vi "Arduino read multiple frequencies.vi"(7 "openQCM gate time":i32, 8 "arduino addresses in":T1, 11 "arduinos on?":bool) -> (0 "arduino addresses out":T1, 1 "openQCM frequencies out":T2, 3 "arduinos on":bool)   [LabVIEW 2014]
uses:
  <vilib>/Analysis/baseanly.llb/Mean (DBL).vi
  <vilib>/Analysis/NI_AALBase.lvlib
panel:
  out "Temp (K) 6":dbl
  out "Temp (K) 5":dbl
  out "Temp (K) 4":dbl
  out "Temp (K) 3":dbl
  out "Temp (K) 2":dbl
  out "Temp (K)":dbl
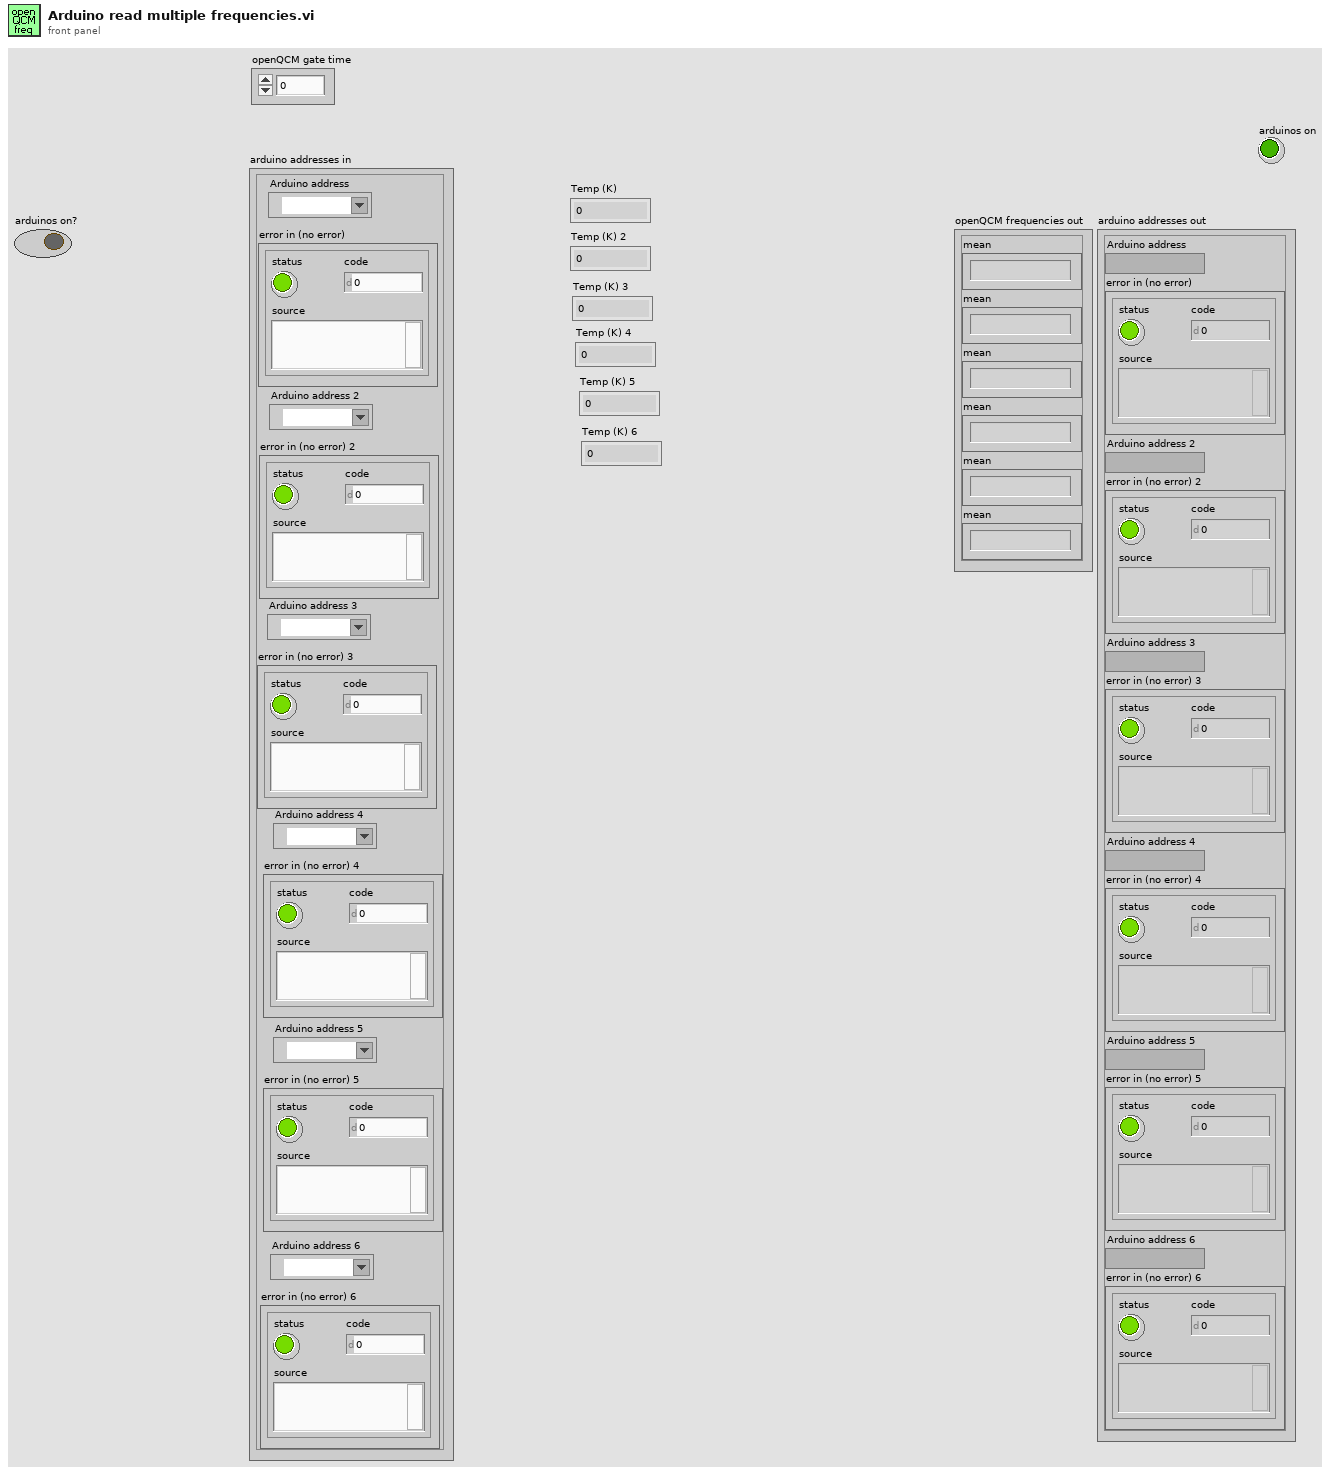
[diagram p1: front panel]
types:
  T1 = cluster{"Arduino address":refnum<visa-resource-name>, "error in (no error)":errorcluster, "Arduino address 2":refnum<visa-resource-name>, "error in (no error) 2":errorcluster, "Arduino address 3":refnum<visa-resource-name>, "error in (no error) 3":errorcluster, "Arduino address 4":refnum<visa-resource-name>, "error in (no error) 4":errorcluster, "Arduino address 5":refnum<visa-resource-name>, "error in (no error) 5":errorcluster, "Arduino address 6":refnum<visa-resource-name>, "error in (no error) 6":errorcluster}
  T2 = cluster{"mean":string, "mean":string, "mean":string, "mean":string, "mean":string, "mean":string}
  T3 = cluster{"mean":dbl, "mean":dbl, "mean":dbl, "mean":dbl, "mean":dbl, "mean":dbl}
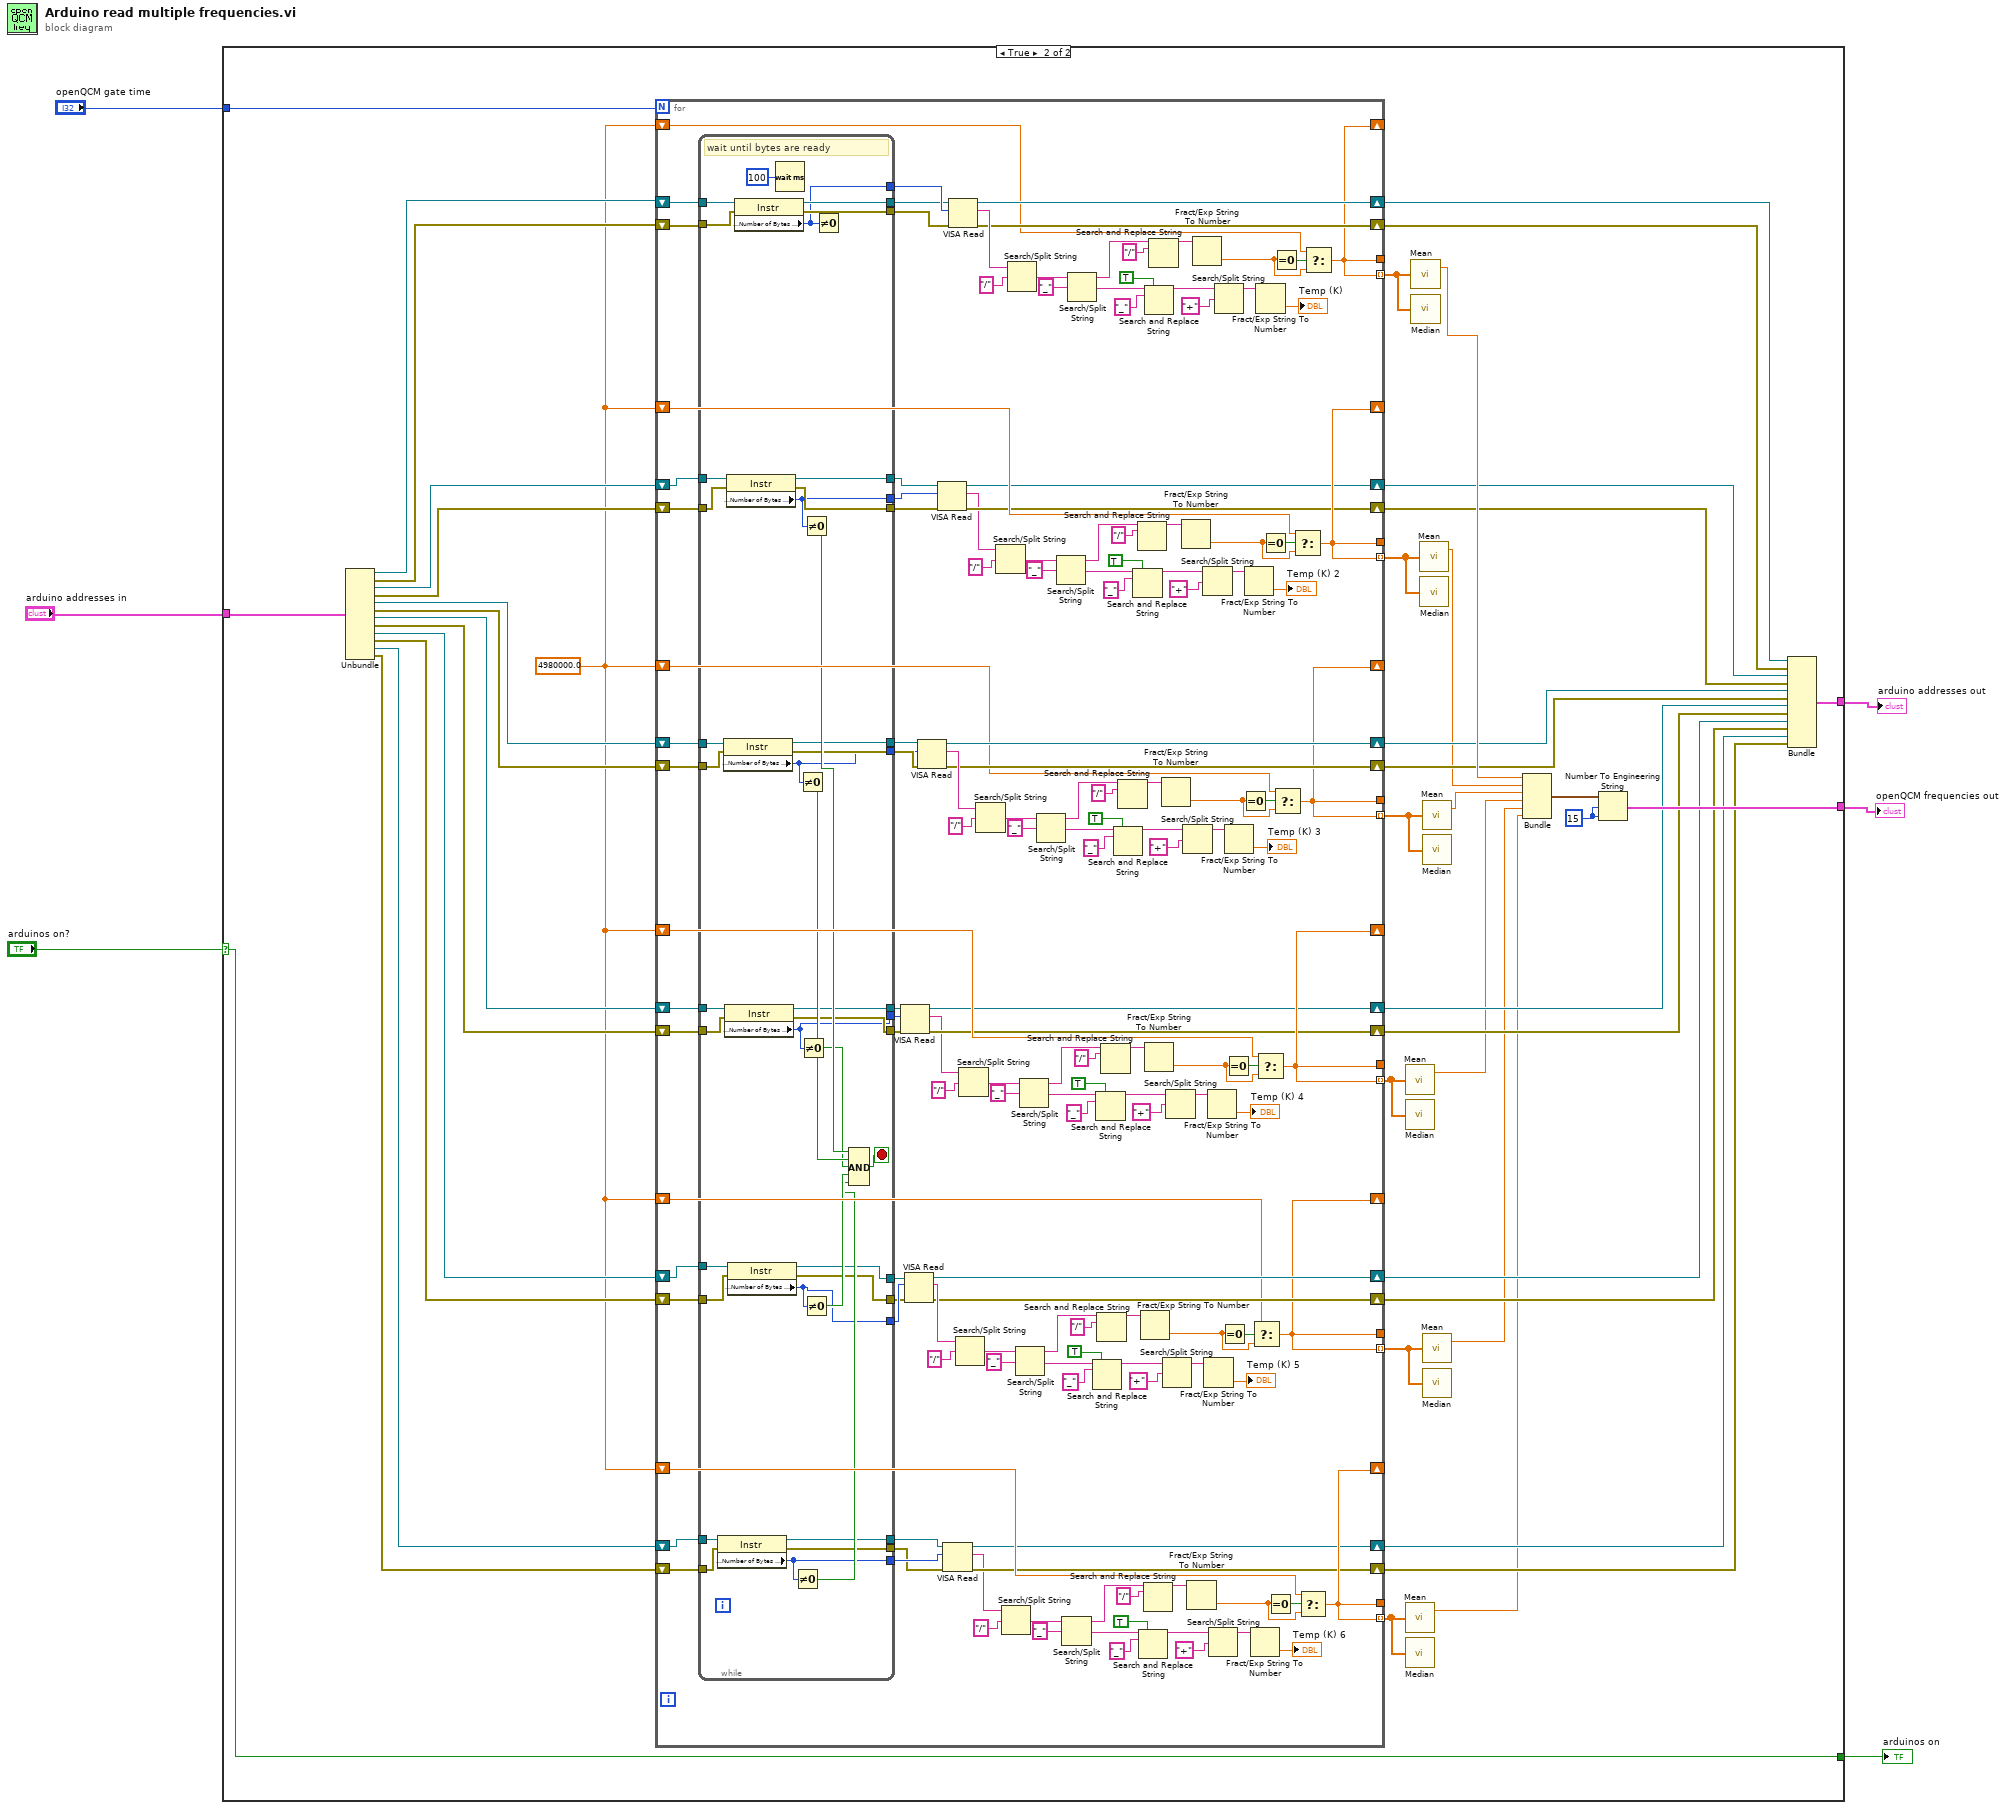
[diagram p0: block diagram]
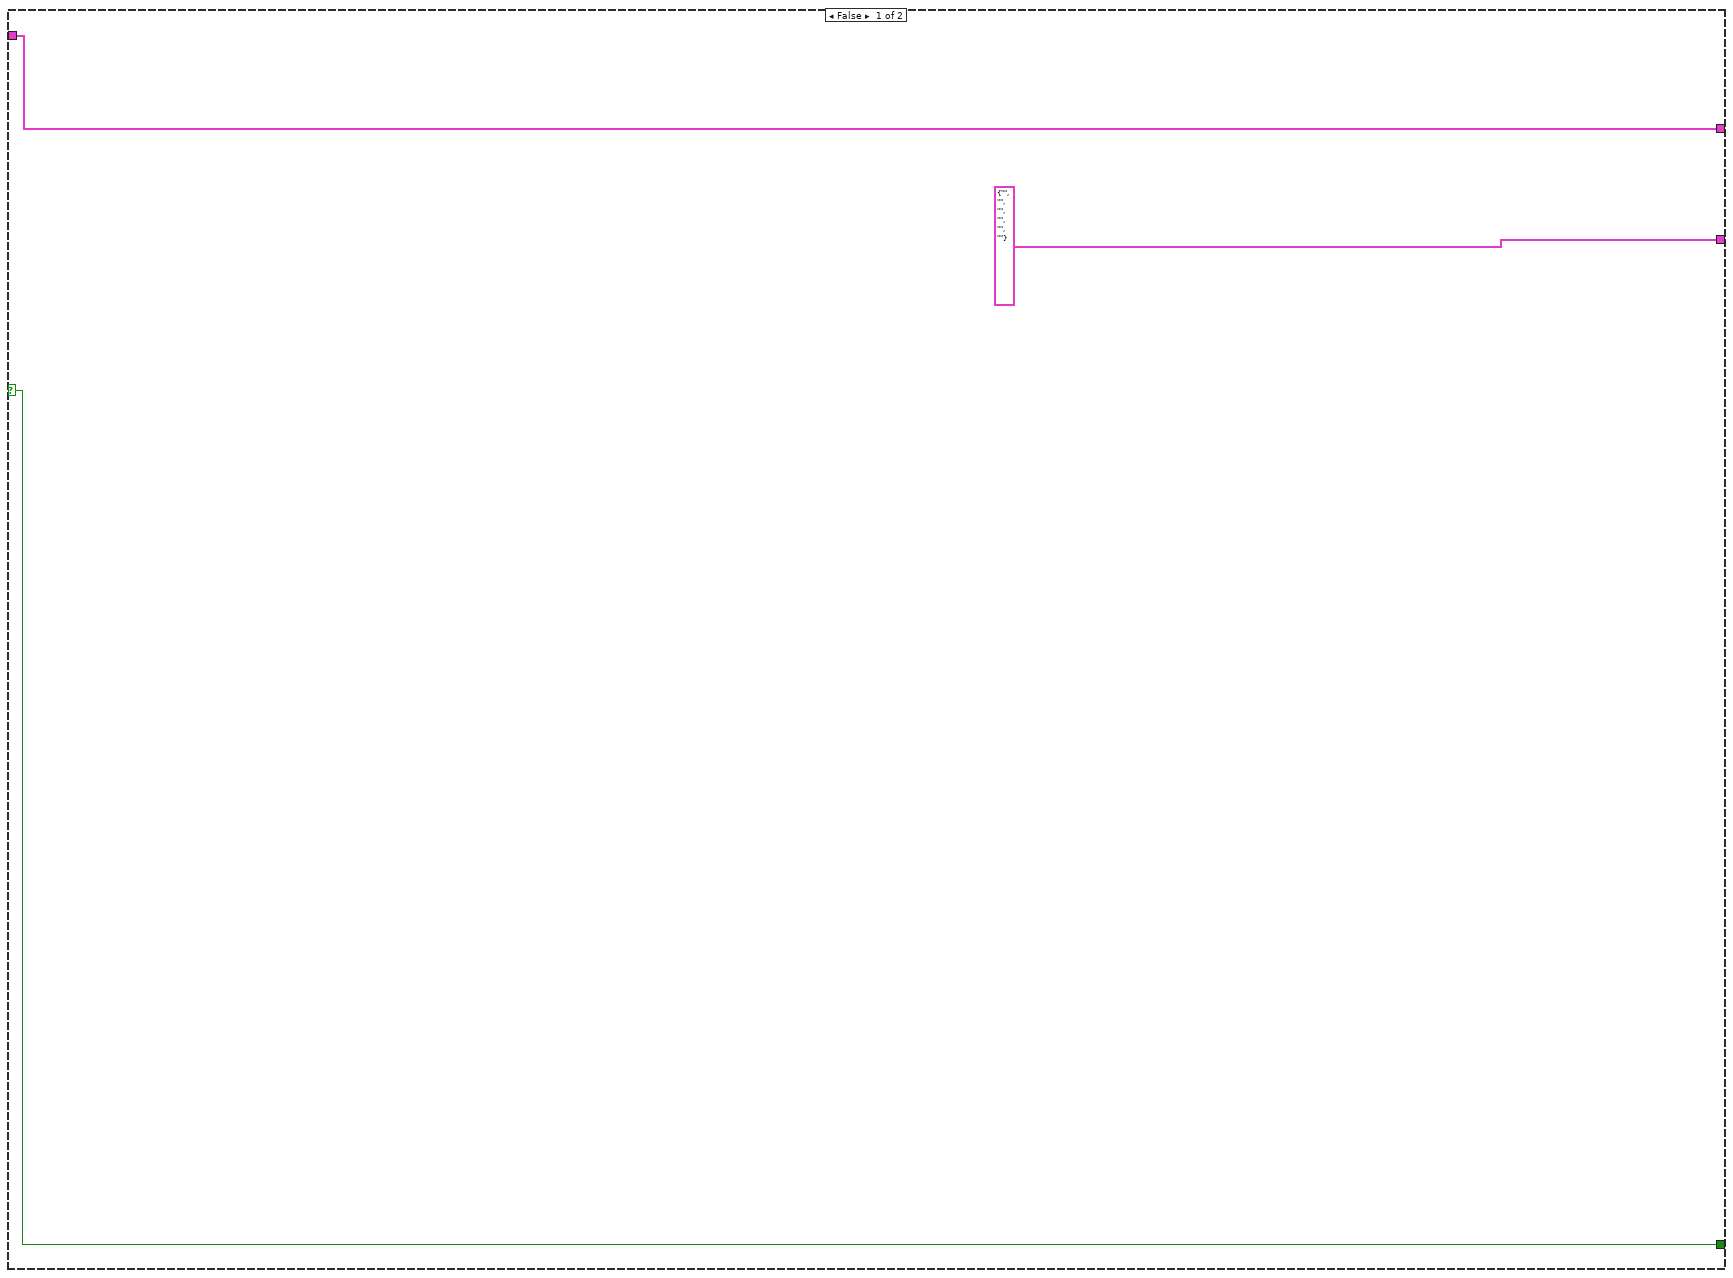
[diagram p2: hidden frame]
diagram:
  n1 = case shown="True" "arduinos on?" {
    selector: "arduinos on?" -> [w9 w10]
    tunnel: "arduino addresses in" -> [w8 w53]
    tunnel: "openQCM gate time" -> [_ w49]
    tunnel: [T2 {"mean"="", "mean"="", "mean"="", "mean"="", "mean"="", "mean"=""} w47] -> w4
    tunnel: [w8 w11] -> w3
    tunnel: [w9 w10] -> w1
    frame False {
    }
    frame True {
      w27 = 4980000.0
      w50 = i16 15 ("width (-)")
      n2 = Unbundle(w53) -> ("Arduino address"=w52:refnum<visa-resource-name>, "error in (no error)"=w51:errorcluster, "Arduino address 2"=w37:refnum<visa-resource-name>, "error in (no error) 2"=w36:errorcluster, "Arduino address 3"=w35:refnum<visa-resource-name>, "error in (no error) 3"=w34:errorcluster, "Arduino address 4"=w33:refnum<visa-resource-name>, "error in (no error) 4"=w32:errorcluster, "Arduino address 5"=w31:refnum<visa-resource-name>, "error in (no error) 5"=w28:errorcluster, "Arduino address 6"=w29:refnum<visa-resource-name>, "error in (no error) 6"=w30:errorcluster)
      n3 = for {
        N: w49 -> [_]
        tunnel: [w180] -> _
        shift-right: [w189] -> w44
        shift-left: w52 -> [w184]
        shift-right: [w188] -> w43
        shift-left: w51 -> [w183]
        tunnel: [w180] -> w48 mode=indexing
        shift-right: [w180] -> _
        shift-left: w27 -> [w179]
        tunnel: [w177] -> _
        shift-right: [w173] -> w26
        shift-left: w37 -> [w78]
        shift-right: [w174] -> w25
        shift-left: w36 -> [w77]
        tunnel: [w177] -> w42 mode=indexing
        shift-right: [w177] -> _
        shift-left: w27 -> [w178]
        tunnel: [w140] -> _
        shift-right: [w144] -> w24
        shift-left: w35 -> [w70]
        shift-right: [w143] -> w23
        shift-left: w34 -> [w69]
        tunnel: [w140] -> w41 mode=indexing
        shift-right: [w140] -> _
        shift-left: w27 -> [w139]
        tunnel: [w137] -> _
        shift-right: [w133] -> w22
        shift-left: w33 -> [w68]
        shift-right: [w134] -> w21
        shift-left: w32 -> [w67]
        tunnel: [w137] -> w40 mode=indexing
        shift-right: [w137] -> _
        shift-left: w27 -> [w138]
        tunnel: [w100] -> _
        shift-right: [w104] -> w20
        shift-left: w31 -> [w59]
        shift-right: [w103] -> w19
        shift-left: w28 -> [w58]
        tunnel: [w100] -> w39 mode=indexing
        shift-right: [w100] -> _
        shift-left: w27 -> [w99]
        tunnel: [w97] -> _
        shift-right: [w93] -> w18
        shift-left: w29 -> [w61]
        shift-right: [w94] -> w17
        shift-left: w30 -> [w60]
        tunnel: [w97] -> w38 mode=indexing
        shift-right: [w97] -> _
        shift-left: w27 -> [w98]
        n4 = while {
          tunnel: w183 -> [w239]
          tunnel: w184 -> [w240]
          tunnel: [w238] -> w182
          tunnel: [w237] -> w181
          tunnel: [w236] -> w185
          tunnel: w78 -> [w232]
          tunnel: w77 -> [w231]
          tunnel: [w230] -> w74
          tunnel: [w229] -> w75
          tunnel: [w228] -> w76
          tunnel: [w227] -> w73
          tunnel: [w226] -> w72
          tunnel: [w225] -> w71
          tunnel: w70 -> [w224]
          tunnel: w69 -> [w223]
          tunnel: w68 -> [w221]
          tunnel: w67 -> [w220]
          tunnel: [w219] -> w54
          tunnel: [w218] -> w66
          tunnel: [w217] -> w65
          tunnel: [w213] -> w64
          tunnel: [w212] -> w63
          tunnel: [w211] -> w62
          tunnel: w61 -> [w210]
          tunnel: w60 -> [w209]
          tunnel: w59 -> [w208]
          tunnel: w58 -> [w207]
          tunnel: [w205] -> w57
          tunnel: [w206] -> w56
          tunnel: [w204] -> w55
          stop <- w233 stop-if-true
          # "wait until bytes are ready"
          n5 = property class="Instr"(reference=w210, error in=w209) -> (reference out=w211:refnum<visa-resource-name>, error out=w212:errorcluster, "Serial Settings:Number of Bytes at Serial Port"=w213:u32)
          n6 = property class="Instr"(reference=w224, error in=w223) -> (reference out=w225:refnum<visa-resource-name>, error out=w227:errorcluster, "Serial Settings:Number of Bytes at Serial Port"=w226:u32)
          n7 = property class="Instr"(reference=w221, error in=w220) -> (reference out=w219:refnum<visa-resource-name>, error out=w218:errorcluster, "Serial Settings:Number of Bytes at Serial Port"=w217:u32)
          n8 = property class="Instr"(reference=w232, error in=w231) -> (reference out=w230:refnum<visa-resource-name>, error out=w229:errorcluster, "Serial Settings:Number of Bytes at Serial Port"=w228:u32)
          n9 = property class="Instr"(reference=w208, error in=w207) -> (reference out=w205:refnum<visa-resource-name>, error out=w204:errorcluster, "Serial Settings:Number of Bytes at Serial Port"=w206:u32)
          n10 = property class="Instr"(reference=w240, error in=w239) -> (reference out=w237:refnum<visa-resource-name>, error out=w238:errorcluster, "Serial Settings:Number of Bytes at Serial Port"=w236:u32)
          n11 = Wait (ms)(milliseconds to wait=u32 100) -> ()  [unwired: 1 out]
          n12 = Not Equal To 0?(x=w213) -> (x != 0?=w214:bool)
          n13 = Not Equal To 0?(x=w226) -> (x != 0?=w222:bool)
          n14 = Not Equal To 0?(x=w217) -> (x != 0?=w216:bool)
          n15 = Not Equal To 0?(x=w228) -> (x != 0?=w234:bool)
          n16 = Not Equal To 0?(x=w206) -> (x != 0?=w215:bool)
          n17 = Not Equal To 0?(x=w236) -> ()  [unwired: 1 out]
          n18 = Compound Arithmetic op=AND(w234, w222, w216, w215, w214) -> (w233:bool)
        }
        n19 = VISA Read(VISA resource name=w54, byte count=w65, error in (no error)=w66) -> (VISA resource name out=w133:refnum<visa-resource-name>, read buffer=w119:string, error out=w134:errorcluster)  [unwired: 1 out]
        n20 = VISA Read(VISA resource name=w57, byte count=w56, error in (no error)=w55) -> (VISA resource name out=w104:refnum<visa-resource-name>, read buffer=w118:string, error out=w103:errorcluster)  [unwired: 1 out]
        n21 = VISA Read(VISA resource name=w71, byte count=w72, error in (no error)=w73) -> (VISA resource name out=w144:refnum<visa-resource-name>, read buffer=w158:string, error out=w143:errorcluster)  [unwired: 1 out]
        n22 = VISA Read(VISA resource name=w74, byte count=w76, error in (no error)=w75) -> (VISA resource name out=w173:refnum<visa-resource-name>, read buffer=w159:string, error out=w174:errorcluster)  [unwired: 1 out]
        n23 = VISA Read(VISA resource name=w62, byte count=w64, error in (no error)=w63) -> (VISA resource name out=w93:refnum<visa-resource-name>, read buffer=w79:string, error out=w94:errorcluster)  [unwired: 1 out]
        n24 = VISA Read(VISA resource name=w181, byte count=w185, error in (no error)=w182) -> (VISA resource name out=w189:refnum<visa-resource-name>, read buffer=w203:string, error out=w188:errorcluster)  [unwired: 1 out]
        n25 = Search/Split String(string=w118, search string/char (-)="/") -> (match + rest of string=w110:string)  [unwired: 1 in, 2 out]
        n26 = Search/Split String(string=w119, search string/char (-)="/") -> (match + rest of string=w127:string)  [unwired: 1 in, 2 out]
        n27 = Search/Split String(string=w158, search string/char (-)="/") -> (match + rest of string=w150:string)  [unwired: 1 in, 2 out]
        n28 = Search/Split String(string=w159, search string/char (-)="/") -> (match + rest of string=w167:string)  [unwired: 1 in, 2 out]
        n29 = Search/Split String(string=w79, search string/char (-)="/") -> (match + rest of string=w87:string)  [unwired: 1 in, 2 out]
        n30 = Search/Split String(string=w203, search string/char (-)="/") -> (match + rest of string=w195:string)  [unwired: 1 in, 2 out]
        n31 = Search/Split String(string=w110, search string/char (-)="_") -> (substring before match=w116:string, match + rest of string=w111:string)  [unwired: 1 in, 1 out]
        n32 = Search/Split String(string=w127, search string/char (-)="_") -> (substring before match=w121:string, match + rest of string=w126:string)  [unwired: 1 in, 1 out]
        n33 = Search/Split String(string=w150, search string/char (-)="_") -> (substring before match=w156:string, match + rest of string=w151:string)  [unwired: 1 in, 1 out]
        n34 = Search/Split String(string=w167, search string/char (-)="_") -> (substring before match=w161:string, match + rest of string=w166:string)  [unwired: 1 in, 1 out]
        n35 = Search/Split String(string=w87, search string/char (-)="_") -> (substring before match=w81:string, match + rest of string=w86:string)  [unwired: 1 in, 1 out]
        n36 = Search/Split String(string=w195, search string/char (-)="_") -> (substring before match=w201:string, match + rest of string=w196:string)  [unwired: 1 in, 1 out]
        n37 = Search and Replace String(replace all?=TRUE ("replace all? (F)"), input string=w111, search string="_") -> (result string=w105:string)  [unwired: 5 in, 3 out]
        n38 = Search and Replace String(replace all?=TRUE ("replace all? (F)"), input string=w126, search string="_") -> (result string=w132:string)  [unwired: 5 in, 3 out]
        n39 = Search and Replace String(input string=w116, search string="/" ("replace string (\"\")")) -> (result string=w107:string)  [unwired: 6 in, 3 out]
        n40 = Search and Replace String(input string=w121, search string="/" ("replace string (\"\")")) -> (result string=w130:string)  [unwired: 6 in, 3 out]
        n41 = Search and Replace String(replace all?=TRUE ("replace all? (F)"), input string=w151, search string="_") -> (result string=w145:string)  [unwired: 5 in, 3 out]
        n42 = Search and Replace String(input string=w156, search string="/" ("replace string (\"\")")) -> (result string=w147:string)  [unwired: 6 in, 3 out]
        n43 = Search and Replace String(replace all?=TRUE ("replace all? (F)"), input string=w166, search string="_") -> (result string=w172:string)  [unwired: 5 in, 3 out]
        n44 = Search and Replace String(input string=w161, search string="/" ("replace string (\"\")")) -> (result string=w170:string)  [unwired: 6 in, 3 out]
        n45 = Search and Replace String(replace all?=TRUE ("replace all? (F)"), input string=w86, search string="_") -> (result string=w92:string)  [unwired: 5 in, 3 out]
        n46 = Fract/Exp String To Number(string=w107) -> (number=w101:dbl)  [unwired: 3 in, 1 out]
        n47 = Search and Replace String(input string=w81, search string="/" ("replace string (\"\")")) -> (result string=w90:string)  [unwired: 6 in, 3 out]
        n48 = Search and Replace String(replace all?=TRUE ("replace all? (F)"), input string=w196, search string="_") -> (result string=w190:string)  [unwired: 5 in, 3 out]
        n49 = Fract/Exp String To Number(string=w130) -> (number=w136:dbl)  [unwired: 3 in, 1 out]
        n50 = Search and Replace String(input string=w201, search string="/" ("replace string (\"\")")) -> (result string=w192:string)  [unwired: 6 in, 3 out]
        n51 = Fract/Exp String To Number(string=w147) -> (number=w141:dbl)  [unwired: 3 in, 1 out]
        n52 = Search/Split String(string=w105, search string/char (-)="+") -> (substring before match=w114:string)  [unwired: 1 in, 2 out]
        n53 = Search/Split String(string=w132, search string/char (-)="+") -> (substring before match=w123:string)  [unwired: 1 in, 2 out]
        n54 = Fract/Exp String To Number(string=w170) -> (number=w176:dbl)  [unwired: 3 in, 1 out]
        n55 = Search/Split String(string=w145, search string/char (-)="+") -> (substring before match=w154:string)  [unwired: 1 in, 2 out]
        n56 = Fract/Exp String To Number(string=w90) -> (number=w96:dbl)  [unwired: 3 in, 1 out]
        n57 = Fract/Exp String To Number(string=w192) -> (number=w186:dbl)  [unwired: 3 in, 1 out]
        n58 = Search/Split String(string=w172, search string/char (-)="+") -> (substring before match=w163:string)  [unwired: 1 in, 2 out]
        n59 = Fract/Exp String To Number(string=w114) -> (number=→"Temp (K) 5":dbl)  [unwired: 3 in, 1 out]
        n60 = Fract/Exp String To Number(string=w123) -> (number=→"Temp (K) 4":dbl)  [unwired: 3 in, 1 out]
        n61 = Search/Split String(string=w92, search string/char (-)="+") -> (substring before match=w83:string)  [unwired: 1 in, 2 out]
        n62 = Search/Split String(string=w190, search string/char (-)="+") -> (substring before match=w199:string)  [unwired: 1 in, 2 out]
        n63 = Equal To 0?(x=w101) -> (x = 0?=w102:bool)
        n64 = Equal To 0?(x=w136) -> (x = 0?=w135:bool)
        n65 = Fract/Exp String To Number(string=w154) -> (number=→"Temp (K) 3":dbl)  [unwired: 3 in, 1 out]
        n66 = Equal To 0?(x=w141) -> (x = 0?=w142:bool)
        n67 = Fract/Exp String To Number(string=w163) -> (number=→"Temp (K) 2":dbl)  [unwired: 3 in, 1 out]
        n68 = Fract/Exp String To Number(string=w83) -> (number=→"Temp (K) 6":dbl)  [unwired: 3 in, 1 out]
        n69 = Select(t=w99, s=w102, f=w101) -> (s? t:f=w100:dbl)
        n70 = Fract/Exp String To Number(string=w199) -> (number=→"Temp (K)":dbl)  [unwired: 3 in, 1 out]
        n71 = Select(t=w138, s=w135, f=w136) -> (s? t:f=w137:dbl)
        n72 = Equal To 0?(x=w176) -> (x = 0?=w175:bool)
        n73 = Equal To 0?(x=w96) -> (x = 0?=w95:bool)
        n74 = Equal To 0?(x=w186) -> (x = 0?=w187:bool)
        n75 = Select(t=w139, s=w142, f=w141) -> (s? t:f=w140:dbl)
        n76 = Select(t=w178, s=w175, f=w176) -> (s? t:f=w177:dbl)
        n77 = Select(t=w98, s=w95, f=w96) -> (s? t:f=w97:dbl)
        n78 = Select(t=w179, s=w187, f=w186) -> (s? t:f=w180:dbl)
      }
      n79 = call-poly <vilib>:"Mean.vi"("X"=w40) -> ("mean"=w14:dbl)  [unwired: 1 out]
      n80 = call <vilib>:"Median.vi"("X"=w40) -> ()  [unwired: 2 out]
      n81 = call-poly <vilib>:"Mean.vi"("X"=w38) -> ("mean"=w12:dbl)  [unwired: 1 out]
      n82 = call <vilib>:"Median.vi"("X"=w38) -> ()  [unwired: 2 out]
      n83 = call-poly <vilib>:"Mean.vi"("X"=w48) -> ("mean"=w46:dbl)  [unwired: 1 out]
      n84 = call <vilib>:"Median.vi"("X"=w48) -> ()  [unwired: 2 out]
      n85 = call-poly <vilib>:"Mean.vi"("X"=w42) -> ("mean"=w16:dbl)  [unwired: 1 out]
      n86 = call <vilib>:"Median.vi"("X"=w42) -> ()  [unwired: 2 out]
      n87 = call-poly <vilib>:"Mean.vi"("X"=w41) -> ("mean"=w15:dbl)  [unwired: 1 out]
      n88 = call <vilib>:"Median.vi"("X"=w41) -> ()  [unwired: 2 out]
      n89 = call-poly <vilib>:"Mean.vi"("X"=w39) -> ("mean"=w13:dbl)  [unwired: 1 out]
      n90 = call <vilib>:"Median.vi"("X"=w39) -> ()  [unwired: 2 out]
      n91 = Bundle("mean"=w46, "mean"=w16, "mean"=w15, "mean"=w14, "mean"=w13, "mean"=w12) -> (w45:T3)  [unwired: 1 in]
      n92 = Number To Engineering String(2:w50, 3:w50, 4:w45) -> (0:w47:T2)  [unwired: 1 in]
      n93 = Bundle("Arduino address"=w44, "error in (no error)"=w43, "Arduino address 2"=w26, "error in (no error) 2"=w25, "Arduino address 3"=w24, "error in (no error) 3"=w23, "Arduino address 4"=w22, "error in (no error) 4"=w21, "Arduino address 5"=w20, "error in (no error) 5"=w19, "Arduino address 6"=w18, "error in (no error) 6"=w17) -> (w11:T1)  [unwired: 1 in]
    }
  }
  "openQCM frequencies out" <- w4
  "arduino addresses out" <- w3
  "arduinos on" <- w1
